vi "Post Launch Init.vi"(8 "error in":errorcluster, 11 "Fault Handler in":refnum<class "Fault Handler.lvclass">) -> (0 "error out":errorcluster, 3 "Fault Handler out":refnum<class "Fault Handler.lvclass">, 4 "Events":T1)   [LabVIEW 2023, in "Fault Handler.lvlib" / "Fault Handler.lvclass"]
doc: "This routine reads the warnings and errors logs and updates the errors and warnings indicators on the front panel for a quick reference to the fault and warnings history.\n\nNext the routine registers for events generated by the <b>Engine</b> Events references."
uses:
  Library/Fault Handler.lvclass
  C:/Users/Public/Documents/Development/builds/Engine/Engine.lvlibp/Project/Engine.lvclass
  builds/Engine/Panel.lvlibp/Panel Helper/Panel Events.ctl
  builds/Engine/Panel.lvlibp/Panel Helper/Events.ctl
  builds/Engine/Engine.lvlibp/Custom Controls/Engine Events.ctl
  builds/Engine/Engine.lvlibp/Custom Controls/System Events.ctl
  builds/Engine/Engine.lvlibp/Custom Controls/System Status.ctl
  builds/Engine/Engine.lvlibp/Custom Controls/Manual Events.ctl
  builds/Engine/Engine.lvlibp/Custom Controls/UUT_Events.ctl
  builds/Engine/Engine.lvlibp/Custom Controls/Interface Events.ctl
  builds/Engine/Engine.lvlibp/Accessors/Read Events.vi
  builds/Engine/Panel Manager.lvlibp/Panel Actor/Panel Actor.lvclass
  C:/Users/Public/Documents/Development/builds/Engine/Panel Manager.lvlibp/Panel Actor/Panel Actor.lvclass
  builds/Engine/Panel.lvlibp/Panel Helper/Panel Helper.lvclass
  builds/Engine/Engine.lvlibp/Project/Engine.lvclass
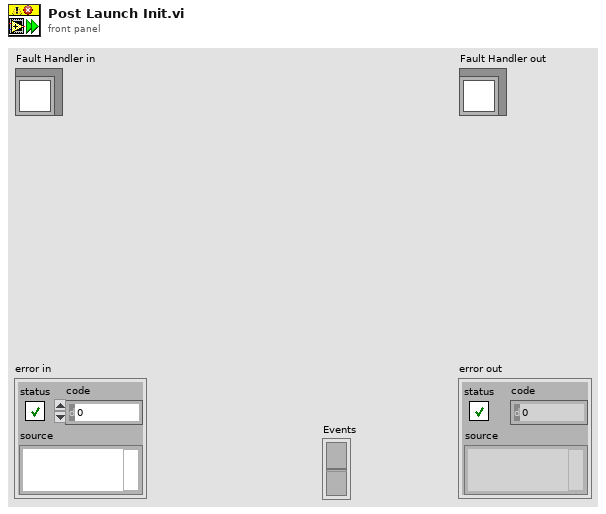
[diagram p1: front panel]
types:
  T1 = cluster{"Pnl Actor":refnum<event-registration>, "Event Registration Refnum":refnum<event-registration>}
  T2 = typedef "Engine.lvlibp/Engine.lvclass/Engine Events.ctl" = cluster{"System Event":T3, "Manual":T4, "UUT":T5, "Interface Events":T6}
  T3 = typedef "Engine.lvlibp/Engine.lvclass/System Events.ctl" = cluster{"Fault Event":refnum<user-event>, "SystemStatus Event":refnum<user-event>, "Automation":refnum<user-event>}
  T4 = typedef "Engine.lvlibp/Engine.lvclass/Manual Events.ctl" = cluster{"QuickStart Event":refnum<user-event>, "SafeBTE Event":refnum<user-event>, "TogglePower Event":refnum<user-event>, "Change Instrument Event":refnum<user-event>, "Toggle Launch Event":refnum<user-event>, "UUTSupply":refnum<user-event>}
  T5 = typedef "Engine.lvlibp/Engine.lvclass/UUT_Events.ctl" = cluster{"UUT_Name":refnum<user-event>, "Test_Name":refnum<user-event>, "Test_Operator":refnum<user-event>, "Test_Witness":refnum<user-event>, "Pedigree_Event":refnum<user-event>}
  T6 = typedef "Engine.lvlibp/Engine.lvclass/Interface Events.ctl" = cluster{"Interface_Command":refnum<user-event>, "Telemetry_Descriptor":refnum<user-event>, "AsynchTLM_Descriptor":refnum<user-event>}
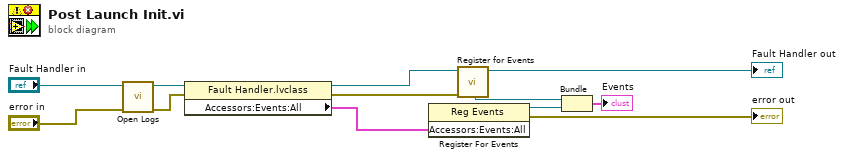
[diagram p0: block diagram]
diagram:
  n1 = call "Open Logs.vi"("error in"="error in", "Fault Handler in"="Fault Handler in") -> ("error out"=w3:errorcluster, "Fault Handler out"=w4:refnum<class "Fault Handler.lvclass">)  [unwired: 8 in]
  n2 = property class="Fault Handler.lvclass"(reference=w4, error in=w3) -> (reference out=w11:refnum<class "Fault Handler.lvclass">, error out=w12:errorcluster, "Accessors:Events:All"=w8:T2)
  n3 = register-events(w8) -> (reference out=w2:refnum<event-registration>, error out=→"error out":errorcluster)  [unwired: 2 in]
  n4 = call "Register for Events.vi"("Error In"=w12, "Panel Actor in"=w11) -> ("Panel Actor out"=→"Fault Handler out":refnum<class "Fault Handler.lvclass">, "Pnl Actor"=w9:refnum<event-registration>)  [unwired: 6 in, 2 out]
  n5 = Bundle("Pnl Actor"=w9, "Event Registration Refnum"=w2) -> (→"Events":T1)  [unwired: 1 in]
